vi "Adjust Coordinate.vi"(9 "Y":dbl, 10 "X":dbl, 11 "Resolution":i32=444) -> (2 "Offset Only":cluster{dbl, dbl}, 3 "Adjusted Coordinate":cluster{dbl, dbl})   [LabVIEW 2013]
doc: "This VI adjusts a coordinate by incorporating the sample size and offset."
uses:
  Global Variables.vi
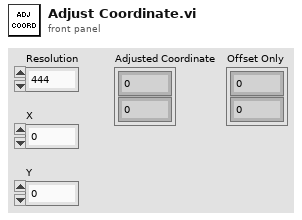
[diagram p1: front panel]
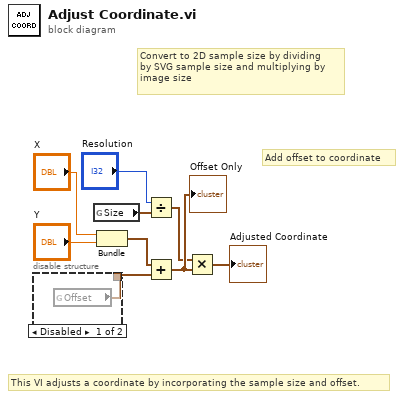
[diagram p0: block diagram]
diagram:
  # "Add offset to coordinate"
  # "Convert to 2D sample size by dividing\nby SVG sample size and multiplying by\nimage size"
  # "This VI adjusts a coordinate by incorporating the sample size and offset."
  n1 = disable-structure shown="Disabled" {
    disable-tunnel: [w10 _] -> w7
    frame Disabled {
      n2 = global read "Global Variables.vi" "Offset"() -> (w10:cluster{"Width":dbl, "Height":dbl})
    }
    frame Enabled {
    }
  }
  n3 = global read "Global Variables.vi" "Size"() -> (w3:cluster{"Width":dbl, "Height":dbl})
  n4 = Bundle("X"="X", "Y"="Y") -> (w8:cluster{"X":dbl, "Y":dbl})  [unwired: 1 in]
  n5 = Divide(x="Resolution", y=w3) -> (x/y=w1:cluster{"Width":dbl, "Height":dbl})
  n6 = Add(x=w8, y=w7) -> (x+y=w9:cluster{dbl, dbl})
  "Offset Only" <- w9
  n7 = Multiply(x=w1, y=w9) -> (x*y=→"Adjusted Coordinate":cluster{dbl, dbl})
